vi "Ask_640_on.vi"(8 "error in":errorcluster, 11 "VISA resource name":refnum<visa-resource-name>) -> (0 "error out":errorcluster, 2 "640 On":bool, 3 "VISA resource name out":refnum<visa-resource-name>)   [LabVIEW 2015]
panel:
  out "Serial Settings:Number of Bytes at Serial Port":u32
  out "read buffer":string
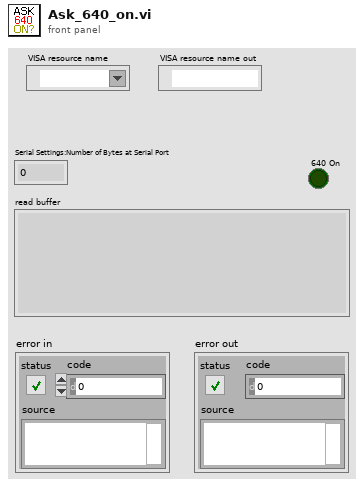
[diagram p1: front panel]
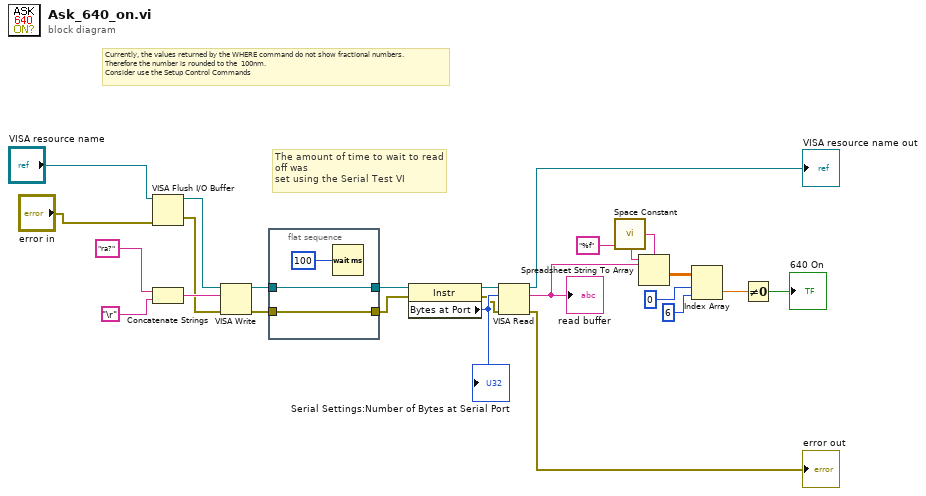
[diagram p0: block diagram]
diagram:
  # "Currently, the values returned by the WHERE command do not show fractional numbers.\nTherefore the number is rounded to the  100nm. \nConsider use the Setup Control Commands"
  # "The amount of time to wait to read off was \nset using the Serial Test VI"
  n1 = VISA Flush I/O Buffer(VISA resource name="VISA resource name", error in (no error)="error in") -> (VISA resource name out=w2:refnum<visa-resource-name>, error out=w1:errorcluster)  [unwired: 1 in]
  n2 = Concatenate Strings("ra?" ("string"), "\r") -> (w15:string)
  n3 = VISA Write(VISA resource name=w2, write buffer=w15, error in (no error)=w1) -> (VISA resource name out=w21:refnum<visa-resource-name>, error out=w19:errorcluster)  [unwired: 1 out]
  n4 = flat-sequence {
    tunnel: [w27] -> w22
    tunnel: w21 -> [w27]
    tunnel: [w25] -> w20
    tunnel: w19 -> [w25]
    frame #0 {
      n5 = Wait (ms)(milliseconds to wait=u32 100) -> ()  [unwired: 1 out]
    }
  }
  n6 = property class="Instr"(reference=w22, error in=w20) -> (reference out=w24:refnum<visa-resource-name>, error out=w18:errorcluster, "Bytes at Port"=w23:u32)
  "Serial Settings:Number of Bytes at Serial Port" <- w23
  n7 = VISA Read(VISA resource name=w24, byte count=w23, error in (no error)=w18) -> (VISA resource name out=→"VISA resource name out":refnum<visa-resource-name>, read buffer=w12:string, error out=→"error out":errorcluster)  [unwired: 1 out]
  "read buffer" <- w12
  n8 = call <vilib>:"Space Constant.vi"() -> ("String"=w11:string)
  n9 = Spreadsheet String To Array(delimiter (Tab)=w11, format string="%f", spreadsheet string=w12) -> (array=w8:dbl[][])  [unwired: 1 in]
  n10 = Index Array(array=w8, index (row)=0, index (col)=6 ("disabled index (col)")) -> (element=w9:dbl)
  n11 = Not Equal To 0?(x=w9) -> (x != 0?=→"640 On":bool)
